vi "Email Global.vi"(7 "Write (F)":bool, 10 "Emails IN":T1[](array[typedef]), 11 "Message IN":string) -> (1 "Emails OUT":T1[](array[typedef]), 2 "Message OUT":string, 3 "Send Email":bool)   [LabVIEW 2020]
uses:
  Type Defs/Email Config.ctl
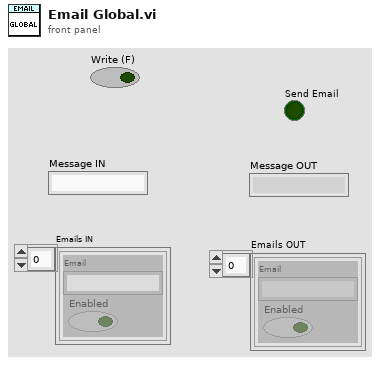
[diagram p1: front panel]
types:
  T1 = typedef "Email Config.ctl" = cluster{"Email":string, "Enabled":bool}
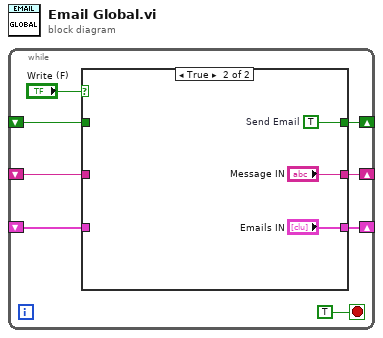
[diagram p0: block diagram]
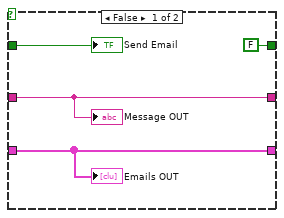
[diagram p2: hidden frame]
diagram:
  n1 = while {
    shift-right: [w6] -> _
    shift-left: _ -> [w5]
    shift-right: [w4] -> _
    shift-left: _ -> [w2]
    shift-right: [w3] -> _
    shift-left: _ -> [w1]
    stop <- TRUE stop-if-true
    n2 = case shown="True" "Write (F)" {
      tunnel: [FALSE ("Send Email") w15] -> w6
      tunnel: w5 -> [w12 _]
      tunnel: [w10 "Message IN"] -> w4
      tunnel: [w9 "Emails IN"] -> w3
      tunnel: w2 -> [w10 _]
      tunnel: w1 -> [w9 _]
      frame False {
        "Send Email" <- w12
        "Message OUT" <- w10
        "Emails OUT" <- w9
      }
      frame True {
        w15 = TRUE  # Send Email
      }
    }
  }
